vi "uTransport_SimpleSend.vi"(5 "Reply CMD (re:<cmd>)":string, 6 "Timestamp (Now)":u32, 7 "Reply Transport":refnum<class "uTransport.lvclass">, 8 "error in (no error)":errorcluster, 9 "Payload":refnum<class "uData.lvclass">, 10 "Msg":string, 11 "uTransport in":refnum<class "uTransport.lvclass">) -> (0 "error out":errorcluster, 3 "uTransport out":refnum<class "uTransport.lvclass">)   [LabVIEW 2021, in "uFramework.lvlib" / "uTransport.lvclass"]
doc: "Simplified method to send a message on a transport. For full control, use the 'Publish' method instead whic is the fully fledged method that allow better messaging scalability."
uses:
  uTransport.lvclass
  Bin/uData.lvlibp/uData.lvclass
  uMsg/uMsg.lvclass/uMsg.ctl
  uMsg/uMsg.lvclass
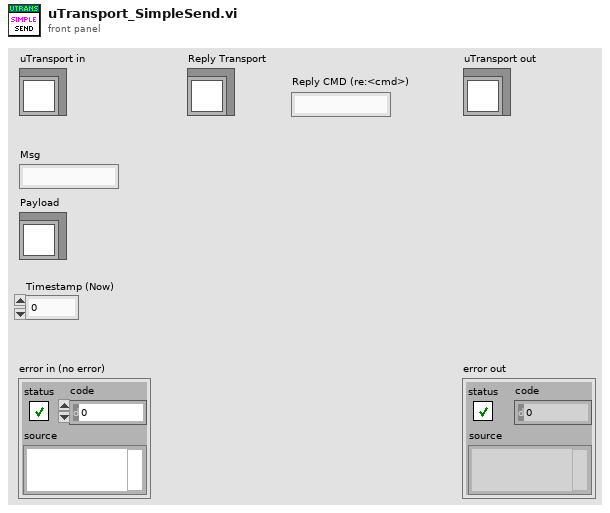
[diagram p1: front panel]
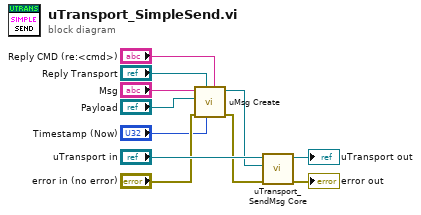
[diagram p0: block diagram]
diagram:
  n1 = call "uMsg Create.vi"("Reply CMD (re:<cmd>)"="Reply CMD (re:<cmd>)", "Timestamp (NULL)"="Timestamp (Now)", "Reply Transport"="Reply Transport", "error in (no error)"="error in (no error)", "Payload"="Payload", "CMD"="Msg") -> ("error out"=w6:errorcluster, "uMsg out"=w8:refnum<class "uMsg.lvclass">)  [unwired: 4 in]
  n2 = call-dynamic "uTransport_SendMsg Core.vi"("error in (no error)"=w6, "Msg"=w8, "uTransport in"="uTransport in") -> ("error out"=→"error out":errorcluster, "uTransport out"=→"uTransport out":refnum<class "uTransport.lvclass">)  [unwired: 7 in]
